vi "Stop_Watch.vi"() -> ()   [LabVIEW 2020]
panel:
  out "sec":dbl max=60.0 step=1.0
  in  "Pause":bool
  out "ms":dbl
  out "min":dbl max=60.0 step=1.0
  out "hour":dbl
  in  "Resume":bool
  in  "Stop":bool
  in  "Reset":bool
  in  "Start":bool
  # "Stop Watch"
  # "INPUT"
  # "OUTPUT"
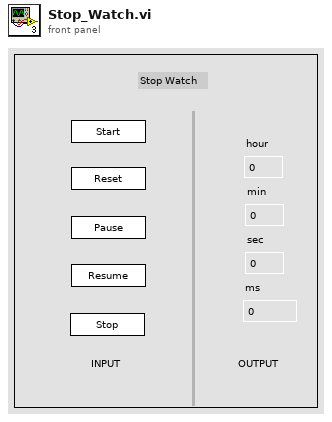
[diagram p1: front panel]
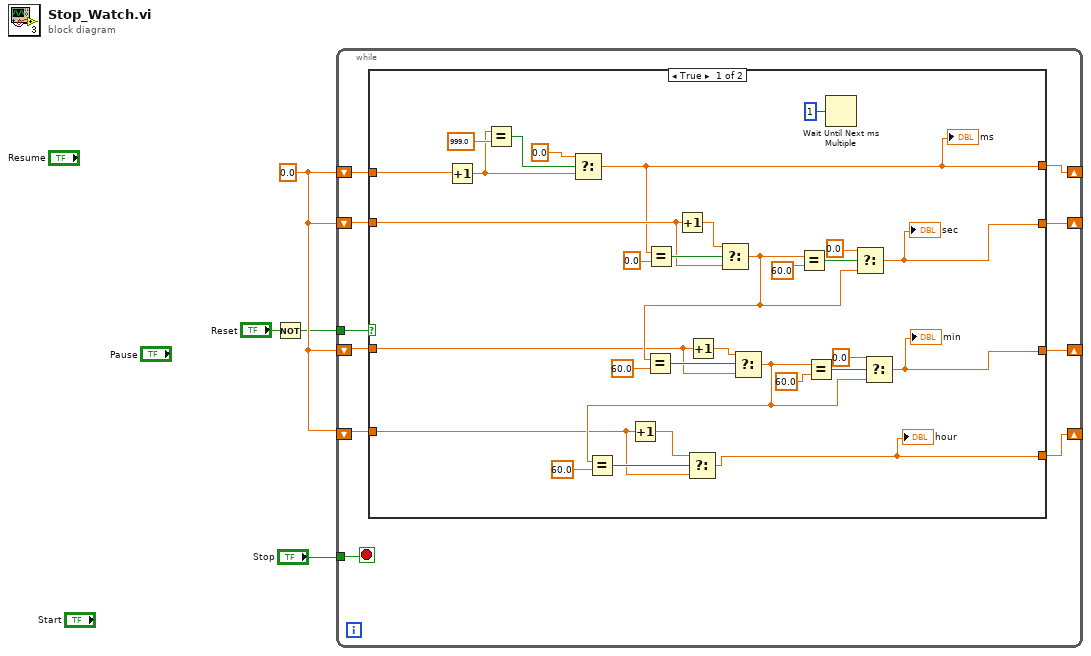
[diagram p0: block diagram]
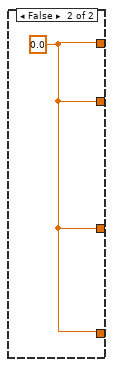
[diagram p2: hidden frame]
diagram:
  w4 = 0.0
  n1 = Not(x="Reset") -> (.not. x?=w2:bool)
  n2 = while {
    shift-right: [w7] -> _
    shift-left: w4 -> [w9]
    shift-right: [w8] -> _
    shift-left: w4 -> [w10]
    shift-right: [w12] -> _
    shift-left: w4 -> [w11]
    shift-right: [w13] -> _
    shift-left: w4 -> [w14]
    tunnel: "Stop" -> [w6]
    tunnel: w2 -> [w5]
    stop <- w6 stop-if-true
    n3 = case shown="True" w5 {
      tunnel: w14 -> [w23 _]
      tunnel: [w15 w45] -> w13
      tunnel: [w16 w45] -> w12
      tunnel: w11 -> [w22 _]
      tunnel: w10 -> [w21 _]
      tunnel: w9 -> [w20 _]
      tunnel: [w17 w45] -> w8
      tunnel: [w18 w45] -> w7
      frame True {
        n4 = Increment(x=w20) -> (x+1=w19:dbl)
        n5 = Equal?(x=w19, y=999.0) -> (x = y?=w42:bool)
        n6 = Select(t=0.0 ("y"), s=w42, f=w19) -> (s? t:f=w18:dbl)
        "ms" <- w18
        n7 = Increment(x=w23) -> (x+1=w29:dbl)
        n8 = Equal?(x=w18, y=0.0) -> (x = y?=w40:bool)
        n9 = Increment(x=w21) -> (x+1=w37:dbl)
        n10 = Increment(x=w22) -> (x+1=w36:dbl)
        n11 = Select(t=w37, s=w40, f=w21) -> (s? t:f=w25:dbl)
        n12 = Equal?(x=w25, y=60.0) -> (x = y?=w34:bool)
        n13 = Select(t=w36, s=w34, f=w22) -> (s? t:f=w24:dbl)
        n14 = Equal?(x=w24, y=60.0) -> (x = y?=w38:bool)
        n15 = Select(t=w29, s=w38, f=w23) -> (s? t:f=w15:dbl)
        "hour" <- w15
        n16 = Equal?(x=w25, y=60.0) -> (x = y?=w32:bool)
        n17 = Equal?(x=w24, y=60.0) -> (x = y?=w27:bool)
        n18 = Wait Until Next ms Multiple(millisecond multiple=u32 1) -> ()  [unwired: 1 out]
        n19 = Select(t=0.0, s=w32, f=w25) -> (s? t:f=w17:dbl)
        "sec" <- w17
        n20 = Select(t=0.0, s=w27, f=w24) -> (s? t:f=w16:dbl)
        "min" <- w16
      }
      frame False {
        w45 = 0.0
      }
    }
  }
